vi "Write Digital Output Status.vi"(8 "error in (no error)":errorcluster, 11 "PXI6521 in":refnum<class "PXI6521.lvclass">) -> (0 "error out":errorcluster, 3 "PXI6521 out":refnum<class "PXI6521.lvclass">)   [LabVIEW 2018, in "PXI6521.lvlib" / "PXI6521.lvclass"]
uses:
  PXI6521.lvclass
  Custom Controls/DAQmx Lines Scope.ctl
  Custom Controls/DAQmx Digital Scope.ctl
  PXI6521.lvclass/PXI6521.ctl
  <vilib>/DAQmx/write.llb/DAQmx Write (Digital 1D Bool 1Chan 1Samp).vi
  <vilib>/DAQmx/create/channels.llb/DAQmx Create Channel (DO-Digital Output).vi
  <vilib>/DAQmx/miscellaneous.llb/DAQmx Fill In Error Info.vi
  PPLs/DigitalIO/Parent/DigitalIO.lvlibp/DigitalIO.lvclass
  PPLs/DigitalIO/Parent/Light Stack.lvlibp/Light Stack.lvclass
  C:/Projects/LabVIEW/PPLs/DigitalIO/Parent/DigitalIO.lvlibp/DigitalIO.lvclass
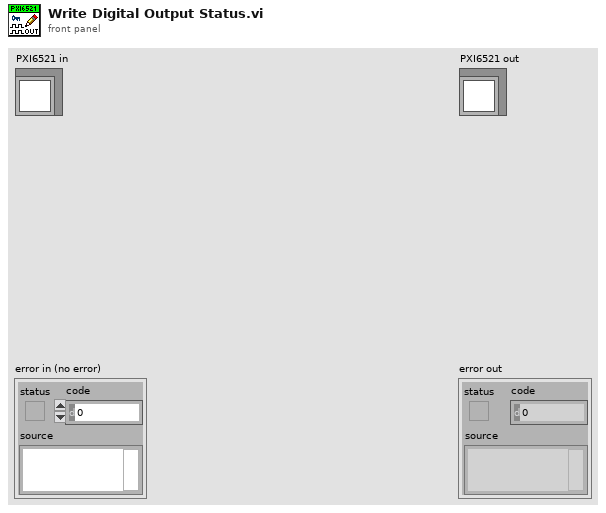
[diagram p1: front panel]
types:
  T1 = typedef "PXI6521.lvlib/PXI6521.lvclass/DAQmx Digital Scope.ctl" = enum16{"Input", "Output"}
  T2 = typedef "PXI6521.lvlib/PXI6521.lvclass/DAQmx Lines Scope.ctl" = enum16{"Full Range", "Custom Range", "Single"}
  T3 = typedef "Light Stack.lvlibp/Light Mode.ctl" = enum16{"OFF", "ON", "BLINK"}
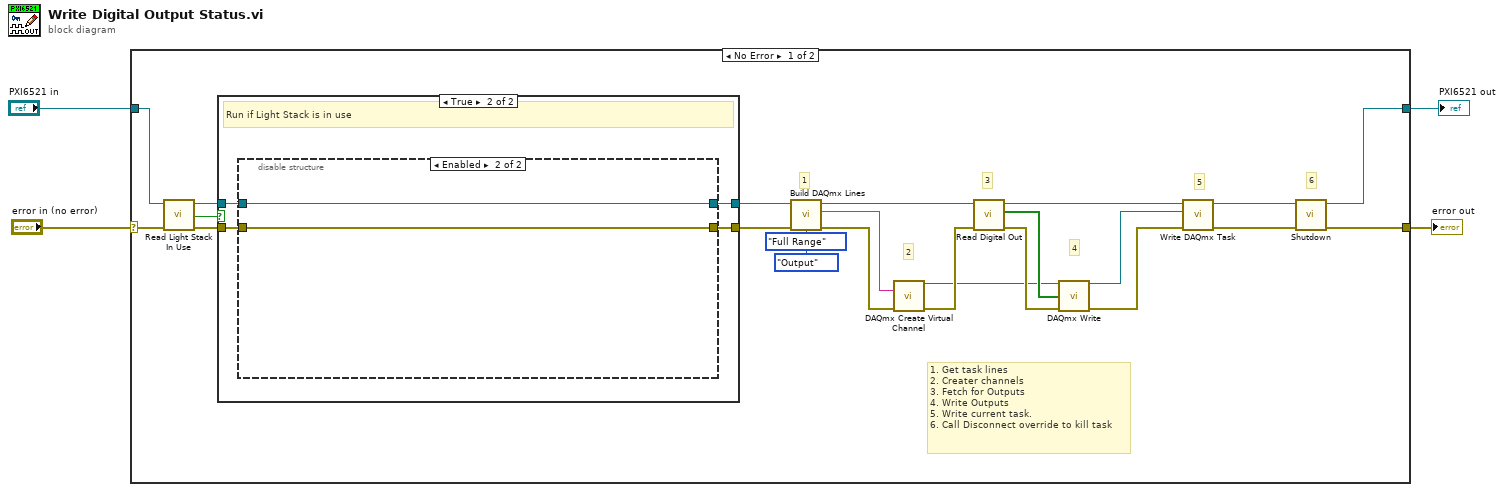
[diagram p0: block diagram]
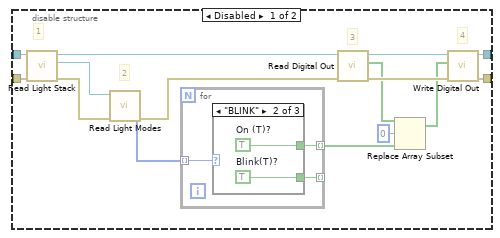
[diagram p3: hidden frame]
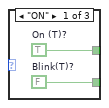
[diagram p4: hidden frame]
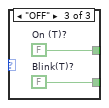
[diagram p5: hidden frame]
diagram:
  n1 = case shown="No Error" "error in (no error)" {
    selector: "error in (no error)" -> [w17 w61]
    tunnel: [w5 w61] -> w3
    tunnel: [w6 w60] -> w1
    tunnel: "PXI6521 in" -> [w16 w60]
    frame No Error {
      # "6"
      # "1. Get task lines\n2. Creater channels\n3. Fetch for Outputs\n4. Write Outputs\n5. Write current task.\n6. Call Disconnect override to kill task"
      # "5"
      # "3"
      # "1"
      # "4"
      # "2"
      n2 = call "Read Light Stack In Use.vi"("error in (no error)"=w17, "DigitalIO in"=w16) -> ("error out"=w18:errorcluster, "Light Stack In Use?"=w20:bool, "DigitalIO out"=w19:refnum<class "PXI6521.lvclass">)  [unwired: 7 in]
      n3 = case shown="True" w20 {
        tunnel: [w29 w30] -> w22
        tunnel: [w28 w31] -> w21
        tunnel: w18 -> [w29 w33]
        tunnel: w19 -> [w28 w32]
        frame False {
          # "Do nothing if Light Stackis not in use"
        }
        frame True {
          # "Run if Light Stack is in use"
          n4 = disable-structure shown="Enabled" {
            disable-tunnel: w33 -> [w45 w58]
            disable-tunnel: w32 -> [w44 w59]
            disable-tunnel: [w35 w59] -> w31
            disable-tunnel: [w34 w58] -> w30
            frame Disabled {
              # "4"
              # "3"
              # "2"
              # "1"
              n5 = call "Read Light Stack.vi"("error in (no error)"=w45, "DigitalIO in"=w44) -> ("error out"=w47:errorcluster, "Light Stack"=w48:refnum<class "Light Stack.lvclass">, "DigitalIO out"=w37:refnum<class "PXI6521.lvclass">)  [unwired: 7 in]
              n6 = call "Read Light Modes.vi"("error in (no error)"=w47, "Light Stack in"=w48) -> ("error out"=w38:errorcluster, "Light Modes"=w46:T3[])  [unwired: 7 in, 1 out]
              n7 = for {
                tunnel: w46 -> [w51] mode=indexing
                tunnel: [w50] -> w36 mode=indexing
                tunnel: [w49] -> _ mode=indexing
                n8 = case shown="\"BLINK\"" w51 {
                  tunnel: [w53 w55 w57] -> w50
                  tunnel: [w52 w54 w56] -> w49
                  frame "ON" {
                    w52 = FALSE  # Blink(T)?
                    w53 = TRUE  # On (T)?
                  }
                  frame "BLINK" {
                    w54 = TRUE  # Blink(T)?
                    w55 = TRUE  # On (T)?
                  }
                  frame "OFF" {
                    w56 = FALSE  # Blink(T)?
                    w57 = FALSE  # On (T)?
                  }
                }
              }
              n9 = call "Read Digital Out.vi"("error in (no error)"=w38, "DigitalIO in"=w37) -> ("error out"=w43:errorcluster, "Digital Out"=w40:bool[], "DigitalIO out"=w41:refnum<class "PXI6521.lvclass">)  [unwired: 7 in]
              n10 = Replace Array Subset(array=w40, new element=w36, index=0) -> (w42:bool[])
              n11 = call "Write Digital Out.vi"("error in (no error)"=w43, "Digital Out"=w42, "DigitalIO in"=w41) -> ("error out"=w34:errorcluster, "DigitalIO out"=w35:refnum<class "PXI6521.lvclass">)  [unwired: 7 in]
            }
            frame Enabled {
            }
          }
        }
      }
      n12 = call "Build DAQmx Lines.vi"("error in (no error)"=w22, "DAQmx Digital Scope"=DAQmx_Digital_Scope."Output", "DAQmx Lines Scope"=DAQmx_Lines_Scope."Full Range", "PXI6521 in"=w21) -> ("error out"=w12:errorcluster, "Full Line"=w24:string, "PXI6521 out"=w13:refnum<class "PXI6521.lvclass">)  [unwired: 5 in]
      n13 = call-poly <vilib>:"DAQmx Create Virtual Channel.vi"("lines"=w24, "error in"=w12) -> ("task out"=w23:refnum<k21>, "error out"=w25:errorcluster)  [unwired: 12 in]
      n14 = call "Read Digital Out.vi"("error in (no error)"=w25, "DigitalIO in"=w13) -> ("error out"=w26:errorcluster, "Digital Out"=w27:bool[], "DigitalIO out"=w9:refnum<class "PXI6521.lvclass">)  [unwired: 7 in]
      n15 = call-poly <vilib>:"DAQmx Write.vi"("task/channels in"=w23, "data"=w27, "error in"=w26) -> ("task out"=w11:refnum<k21>, "error out"=w10:errorcluster)  [unwired: 10 in, 1 out]
      n16 = call "Write DAQmx Task.vi"("error in (no error)"=w10, "DAQmx Task"=w11, "PXI6521 in"=w9) -> ("error out"=w7:errorcluster, "PXI6521 out"=w8:refnum<class "PXI6521.lvclass">)  [unwired: 7 in]
      n17 = call "Shutdown.vi"("error in (no error)"=w7, "DigitalIO in"=w8) -> ("error out"=w5:errorcluster, "DigitalIO out"=w6:refnum<class "PXI6521.lvclass">)  [unwired: 8 in]
    }
    frame Error {
    }
  }
  "error out" <- w3
  "PXI6521 out" <- w1
